vi "Create Trigger Model Log Event Block.vi"(8 "error in (no error)":errorcluster, 9 "Message":string="\"Test\"", 10 "Block Number (1)":i32=1 min=1 format="%#.6g", 11 "VISA resource name":refnum<visa-resource-name>) -> (0 "error out":errorcluster, 3 "VISA resource name out":refnum<visa-resource-name>)   [LabVIEW 2018, in "Keithley DMM7512.lvlib"]
doc: "This VI defines a trigger model block that generates a trigger event and immediately continues to the next block."
uses:
  <instrlib>/Keithley DMM7512/Keithley DMM7512.lvlib
panel:
  in  "Event Type":u16(ring) items=[" Information 1", "Information 2", "Information 3", "Information 4", "Warning 1", "Warning 2", "Warning 3", "Warning 4", "Error 1", "Error 2", "Error 3", "Error 4"]
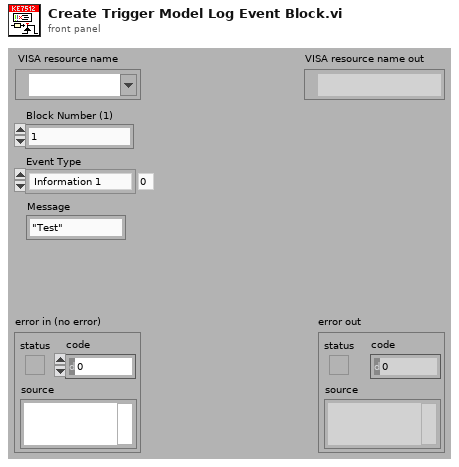
[diagram p1: front panel]
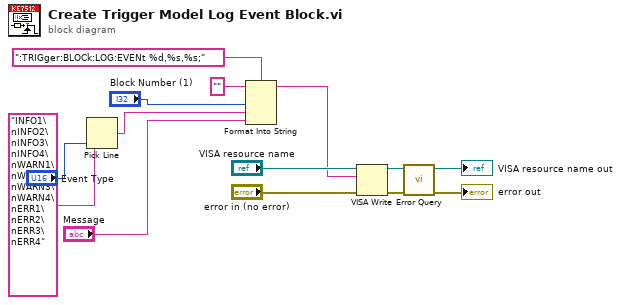
[diagram p0: block diagram]
diagram:
  n1 = Pick Line(multi-line string="INFO1\nINFO2\nINFO3\nINFO4\nWARN1\nWARN2\nWARN3\nWARN4\nERR1\nERR2\nERR3\nERR4", line index="Event Type") -> (output string=w1:string)  [unwired: 1 in]
  n2 = Format Into String(format string=":TRIGger:BLOCk:LOG:EVENt %d,%s,%s;", initial string="", "Block Number (1)", w1, "Message") -> (resulting string=w6:string)  [unwired: 1 in, 1 out]
  n3 = VISA Write(VISA resource name="VISA resource name", write buffer=w6, error in (no error)="error in (no error)") -> (VISA resource name out=w10:refnum<visa-resource-name>, error out=w9:errorcluster)  [unwired: 1 out]
  n4 = call <instrlib>:"Error Query.vi"("error in (no error)"=w9, "VISA resource name"=w10) -> ("error out"=→"error out":errorcluster, "VISA resource name out"=→"VISA resource name out":refnum<visa-resource-name>)  [unwired: 8 out]
